vi "GetFuncIndex.vi"(8 "error in (no error)":errorcluster caption="entrée d'erreur (pas d'erreur)", 11 "Experiment en entrée":refnum<class "Experiment.lvclass"> caption="DNL_LabVIEW Object in") -> (0 "error out":errorcluster caption="sortie d'erreur", 3 "Experiment en sortie":refnum<class "Experiment.lvclass"> caption="DNL_LabVIEW Object out")   [LabVIEW 2019, in "Experiment.lvclass"]
uses:
  Experiment.lvclass
  Experiment.lvclass/Experiment.ctl
  DevicesClass/BaseDevice/BaseDevice.lvclass
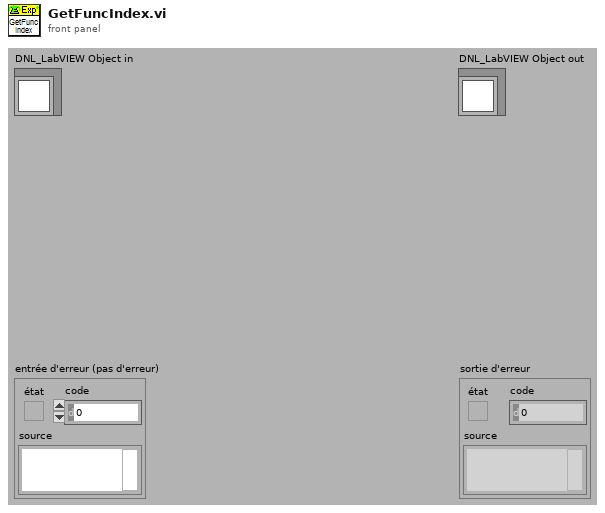
[diagram p1: front panel]
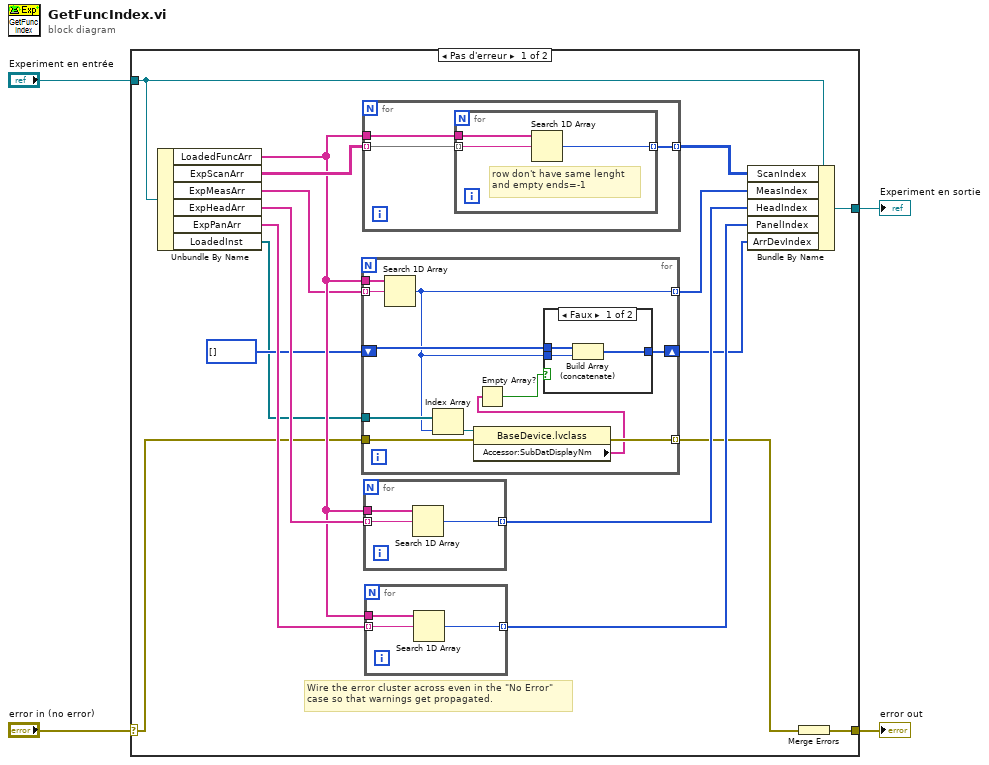
[diagram p0: block diagram]
diagram:
  n1 = case shown="Pas d'erreur" "error in (no error)" {
    selector: "error in (no error)" -> [w8 w50]
    tunnel: [w6 w50] -> w3
    tunnel: [w20 w49] -> w1
    tunnel: "Experiment en entrée" -> [w21 w49]
    frame No Error {
      # "Wire the error cluster across even in the \"No Error\"\ncase so that warnings get propagated."
      n2 = Unbundle By Name(w21) -> ("LoadedFuncArr"=w13:string[], "ExpScanArr"=w19:string[][], "ExpMeasArr"=w5:string[], "ExpHeadArr"=w18:string[], "ExpPanArr"=w12:string[], "LoadedInst"=w9:refnum<class "BaseDevice.lvclass">[])
      n3 = for {
        tunnel: w13 -> [w38]
        tunnel: w5 -> [w37] mode=indexing
        tunnel: [w33] -> w16 mode=indexing
        shift-right: [w35] -> w10
        shift-left: i32[] [] -> [w36]
        tunnel: w9 -> [w34]
        tunnel: w8 -> [w31]
        tunnel: [w30] -> w7 mode=indexing
        n4 = Search 1D Array(1D array=w38, element=w37) -> (index of element=w33:i32)  [unwired: 1 in]
        n5 = Index Array(array=w34, index=w33) -> (element=w32:refnum<class "BaseDevice.lvclass">)
        n6 = property class="BaseDevice.lvclass"(reference=w32, error in=w31) -> (error out=w30:errorcluster, "Accessor:SubDatDisplayNm"=w29:string[])  [unwired: 1 out]
        n7 = Empty Array?(array=w29) -> (empty?=w28:bool)
        n8 = case shown="Faux" w28 {
          tunnel: w36 -> [w41 w42]
          tunnel: [w40 w42] -> w35
          tunnel: w33 -> [w39 _]
          frame False {
            n9 = Build Array (concatenate)(w41, w39) -> (w40:i32[])
          }
          frame True {
          }
        }
      }
      n10 = for {
        tunnel: w13 -> [w45]
        tunnel: w19 -> [w44] mode=indexing
        tunnel: [w43] -> w17 mode=indexing
        n11 = for {
          tunnel: w45 -> [w48]
          tunnel: w44 -> [w47] mode=indexing
          tunnel: [w46] -> w43 mode=indexing
          # "row don't have same lenght\nand empty ends=-1"
          n12 = Search 1D Array(1D array=w48, element=w47) -> (index of element=w46:i32)  [unwired: 1 in]
        }
      }
      n13 = for {
        tunnel: w13 -> [w27]
        tunnel: w18 -> [w26] mode=indexing
        tunnel: [w25] -> w15 mode=indexing
        n14 = Search 1D Array(1D array=w27, element=w26) -> (index of element=w25:i32)  [unwired: 1 in]
      }
      n15 = for {
        tunnel: w13 -> [w24]
        tunnel: w12 -> [w23] mode=indexing
        tunnel: [w22] -> w14 mode=indexing
        n16 = Search 1D Array(1D array=w24, element=w23) -> (index of element=w22:i32)  [unwired: 1 in]
      }
      n17 = Bundle By Name(cluster=w21, "ScanIndex"=w17, "MeasIndex"=w16, "HeadIndex"=w15, "PanelIndex"=w14, "ArrDevIndex"=w10) -> (w20:refnum<class "Experiment.lvclass">)
      n18 = Merge Errors(w7) -> (w6:errorcluster)
    }
    frame Error {
    }
  }
  "error out" <- w3
  "Experiment en sortie" <- w1
